vi "主程序.vi"() -> ()   [LabVIEW 2010]
panel:
  in  "b":dbl
  in  "m":dbl
  in  "x3":dbl
  out "y2":dbl
  out "y":dbl
  in  "x2":dbl
  in  "x":dbl
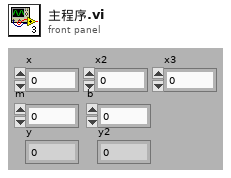
[diagram p1: front panel]
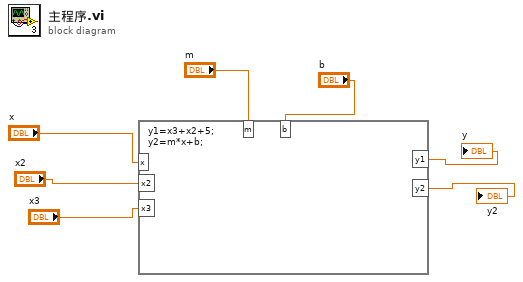
[diagram p0: block diagram]
diagram:
  n1 = formula code="y1=x3+x2+5;\ny2=m*x+b;"("x"="x", "x2"="x2", "x3"="x3", "m"="m", "b"="b") -> ("y1"=→"y":dbl, "y2"=→"y2":dbl)
